vi "Print Error.vi"(7 "error out":errorcluster) -> ()   [LabVIEW 2023, in "NI PXIe-411x PS Custom Device.lvlib"]
uses:
  NI PXIe-411x PS Custom Device.lvlib
  <vilib>/NI VeriStand/Custom Device Tools/Custom Device Utility Library/Custom Device Utility Library.lvlib
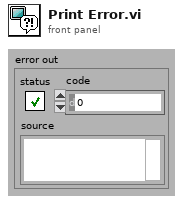
[diagram p1: front panel]
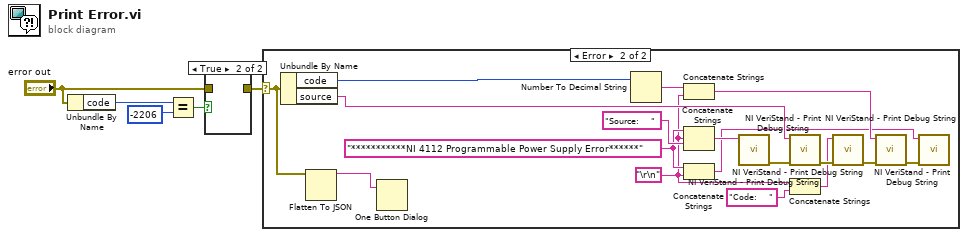
[diagram p0: block diagram]
diagram:
  n1 = Unbundle By Name("error out") -> ("code"=w5:i32)
  n2 = Equal?(x=w5, y=-2206) -> (x = y?=w3:bool)
  n3 = case shown="True" w3 {
    tunnel: "error out" -> [w6 _]
    tunnel: [w6 _] -> w1
    frame False {
    }
    frame True {
    }
  }
  n4 = case shown="Error" w1 {
    selector: w1 -> [_ w8]
    frame No Error {
    }
    frame Error {
      w10 = "\r\n"
      w11 = "***********NI 4112 Programmable Power Supply Error******" ("String")
      n5 = Unbundle By Name(w8) -> ("code"=w20:i32, "source"=w21:string)
      n6 = Flatten To JSON(anything=w8) -> (JSON string=w7:string)  [unwired: 2 in, 1 out]
      n7 = One Button Dialog(message=w7) -> ()  [unwired: 1 in, 1 out]
      n8 = Number To Decimal String(number=w20) -> (decimal integer string=w15:string)  [unwired: 1 in]
      n9 = Concatenate Strings(w15, w10) -> (w14:string)
      n10 = Concatenate Strings(w11, w10, "Source:    " ("String")) -> (w23:string)
      n11 = Concatenate Strings(w11, w10) -> (w9:string)
      n12 = call <vilib>:"NI VeriStand - Print Debug String.vi"("Message"=w23) -> ("error out"=w22:errorcluster)  [unwired: 10 in]
      n13 = call <vilib>:"NI VeriStand - Print Debug String.vi"("error in (no error)"=w22, "Message"=w21) -> ("error out"=w19:errorcluster)  [unwired: 9 in]
      n14 = Concatenate Strings(w10, "Code:    " ("String")) -> (w16:string)
      n15 = call <vilib>:"NI VeriStand - Print Debug String.vi"("error in (no error)"=w19, "Message"=w16) -> ("error out"=w13:errorcluster)  [unwired: 9 in]
      n16 = call <vilib>:"NI VeriStand - Print Debug String.vi"("error in (no error)"=w13, "Message"=w14) -> ("error out"=w12:errorcluster)  [unwired: 9 in]
      n17 = call <vilib>:"NI VeriStand - Print Debug String.vi"("error in (no error)"=w12, "Message"=w9) -> ()  [unwired: 9 in, 1 out]
    }
  }
